vi "Save experiments in PGserver.vi"(6 "Param row name1":string="N", 7 "conninfo":T1={"host"="localhost", "port"="5432", "client_encoding"="WIN1251", "dbname"="system", "user"="postgres", "password"=""}, 8 "error in (no error)":errorcluster, 9 "Param column Name":string="value", 10 "Param Table":string="experiments", 11 "Parameter":string) -> (0 "error out":errorcluster)   [LabVIEW 2019]
uses:
  ctl/Coninfo.ctl
  PostgreSQL2LabVIEW/libpqlv/src/PQresultErrorMessage.vi
  PostgreSQL2LabVIEW/libpqUtility/src/PQclear.vi
  PostgreSQL2LabVIEW/libpqlv/src/PQsendQuery.vi
  PostgreSQL2LabVIEW/libpqlv/src/PQgetResult.vi
  PostgreSQL2LabVIEW/libpqlv/src/PQresultStatus.vi
  PostgreSQL2LabVIEW/libpqlv/src/PQfinish.vi
  PostgreSQL2LabVIEW/libpqlv/src/PQconnectdb.vi
  PostgreSQL2LabVIEW/libpqlv/src/PQerrorMessage.vi
  PostgreSQL2LabVIEW/libpqlv/src/PQstatus.vi
  <vilib>/dlg_ctls.llb/Space Constant.vi
  PostgreSQL2LabVIEW/libpqlv/src/PQclear.vi
  PostgreSQL2LabVIEW/libpqUtility/libpqutility.lvlib
  PostgreSQL2LabVIEW/libpqUtility64/libpqutility64.lvlib
  PostgreSQL.lvlib
panel:
  out "PQStatus":T2(ring)
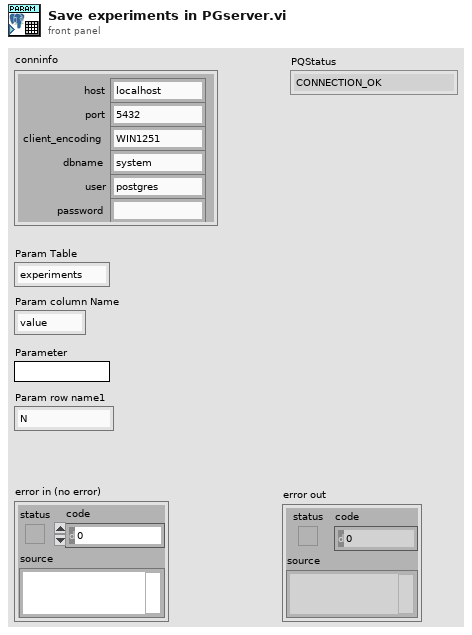
[diagram p1: front panel]
types:
  T1 = typedef "PostgreSQL.lvlib/Coninfo.ctl" = cluster{"host":string, "port":string, "client_encoding":string, "dbname":string, "user":string, "password":string}
  T2 = enum32{"CONNECTION_OK", "CONNECTION_BAD", "CONNECTION_STARTED", "CONNECTION_MADE", "CONNECTION_AWAITING_RESPONSE", "CONNECTION_AUTH_OK", "CONNECTION_SETENV", "CONNECTION_SSL_STARTUP", "CONNECTION_NEEDED"}
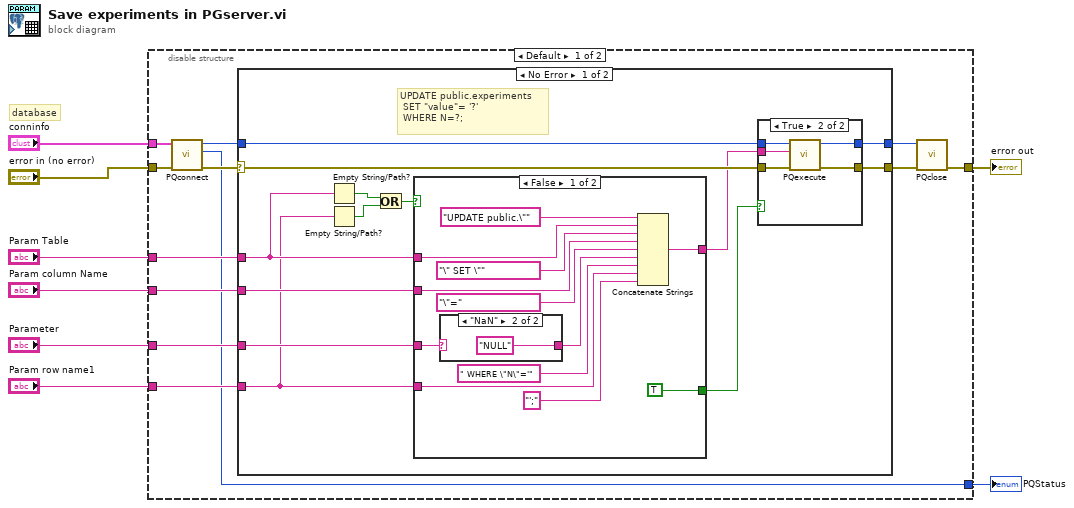
[diagram p0: block diagram]
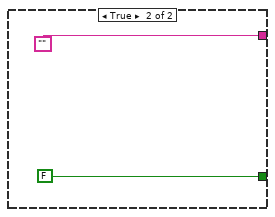
[diagram p3: hidden frame]
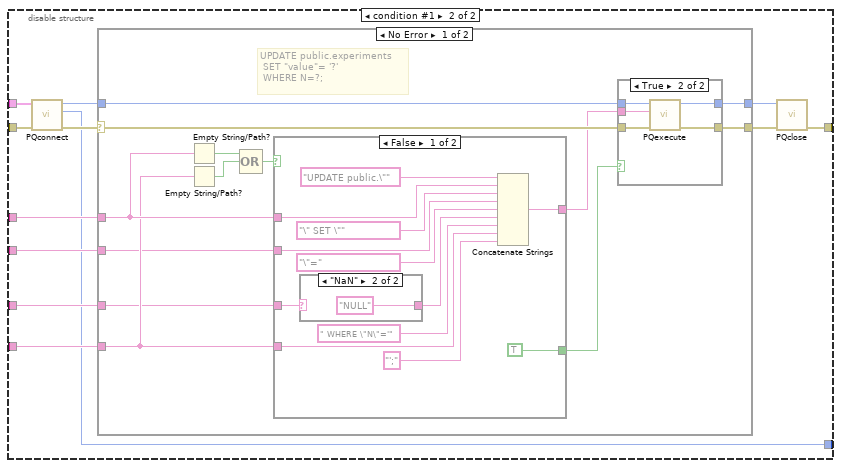
[diagram p6: hidden frame]
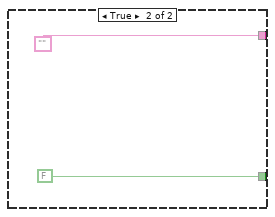
[diagram p8: hidden frame]
diagram:
  # "database"
  n1 = disable-structure shown="Default" {
    disable-tunnel: "Parameter" -> [w18 w62]
    disable-tunnel: [w16 w59] -> w7
    disable-tunnel: "conninfo" -> [w15 w66]
    disable-tunnel: "Param row name1" -> [w13 w61]
    disable-tunnel: "Param Table" -> [w12 w64]
    disable-tunnel: "Param column Name" -> [w11 w63]
    disable-tunnel: "error in (no error)" -> [w10 w65]
    disable-tunnel: [w9 w60] -> w1
    frame condition #0 (active) {
      n2 = call "PQconnect.vi"("error in (no error)"=w10, "conninfo"=w15) -> ("error out"=w20:errorcluster, "PQStatus"=w9:T2, "conn"=w19:u32)  [unwired: 7 in]
      n3 = case shown="No Error" w20 {
        selector: w20 -> [w33 w58]
        tunnel: w18 -> [w27 _]
        tunnel: w19 -> [w32 w57]
        tunnel: w12 -> [w25 _]
        tunnel: [w31 w58] -> w14
        tunnel: w13 -> [w23 _]
        tunnel: w11 -> [w26 _]
        tunnel: [w28 w57] -> w17
        frame No Error {
          # "UPDATE public.experiments\n\tSET \"value\"= '?'\n\tWHERE N=?;"
          n4 = Empty String/Path?(string/path=w25) -> (empty?=w30:bool)
          n5 = Empty String/Path?(string/path=w23) -> (empty?=w29:bool)
          n6 = Or(x=w30, y=w29) -> (x .or. y?=w24:bool)
          n7 = case shown="False" w24 {
            tunnel: [w44 ""] -> w21
            tunnel: w25 -> [w42 _]
            tunnel: [TRUE FALSE] -> w22
            tunnel: w23 -> [w37 _]
            tunnel: w27 -> [w36 _]
            tunnel: w26 -> [w39 _]
            frame False {
              n8 = case shown="\"NaN\"" w36 {
                selector: w36 -> [w46 _]
                tunnel: [w46 "NULL"] -> w35
                frame "", Default {
                }
                frame "NaN" {
                }
              }
              n9 = Concatenate Strings("UPDATE public.\"" ("table"), w42, "\" SET \"" ("table"), w39, "\"=" ("table"), w35, " WHERE \"N\"='" ("string"), w37, "';" ("string")) -> (w44:string)
            }
            frame True {
            }
          }
          n10 = case shown="True" w22 {
            tunnel: w33 -> [w51 w56]
            tunnel: w32 -> [w50 w54]
            tunnel: w21 -> [_ w55]
            tunnel: [w51 w53] -> w31
            tunnel: [w50 w52] -> w28
            frame False {
            }
            frame True {
              n11 = call "PQexecute.vi"("error in"=w56, "SQL querry"=w55, "conn"=w54) -> ("error out"=w53:errorcluster, "conn_out"=w52:u32)  [unwired: 7 in]
            }
          }
        }
        frame Error {
        }
      }
      n12 = call "PQclose.vi"("error in (no error)"=w14, "conn"=w17) -> ("error out"=w16:errorcluster)  [unwired: 9 in]
    }
    frame condition #1 {
      n13 = call "PQconnect.vi"("error in (no error)"=w65, "conninfo"=w66) -> ("error out"=w70:errorcluster, "PQStatus"=w60:T2, "conn"=w69:u64)  [unwired: 7 in]
      n14 = case shown="No Error" w70 {
        selector: w70 -> [w83 w108]
        tunnel: w62 -> [w74 _]
        tunnel: w69 -> [w82 w107]
        tunnel: w64 -> [w77 _]
        tunnel: [w81 w108] -> w67
        tunnel: w61 -> [w75 _]
        tunnel: w63 -> [w73 _]
        tunnel: [w78 w107] -> w68
        frame No Error {
          # "UPDATE public.experiments\n\tSET \"value\"= '?'\n\tWHERE N=?;"
          n15 = Empty String/Path?(string/path=w77) -> (empty?=w80:bool)
          n16 = Empty String/Path?(string/path=w75) -> (empty?=w79:bool)
          n17 = Compound Arithmetic op=OR(w80, w79) -> (w76:bool)  [unwired: 1 in]
          n18 = case shown="False" w76 {
            tunnel: [w94 ""] -> w71
            tunnel: w77 -> [w92 _]
            tunnel: [TRUE FALSE] -> w72
            tunnel: w75 -> [w87 _]
            tunnel: w74 -> [w86 _]
            tunnel: w73 -> [w89 _]
            frame False {
              n19 = case shown="\"NaN\"" w86 {
                selector: w86 -> [w96 _]
                tunnel: [w96 "NULL"] -> w85
                frame "", Default {
                }
                frame "NaN" {
                }
              }
              n20 = Concatenate Strings("UPDATE public.\"" ("table"), w92, "\" SET \"" ("table"), w89, "\"=" ("table"), w85, " WHERE \"N\"='" ("string"), w87, "';" ("string")) -> (w94:string)
            }
            frame True {
            }
          }
          n21 = case shown="True" w72 {
            tunnel: w83 -> [w101 w106]
            tunnel: w82 -> [w100 w104]
            tunnel: w71 -> [_ w105]
            tunnel: [w101 w103] -> w81
            tunnel: [w100 w102] -> w78
            frame False {
            }
            frame True {
              n22 = call "PQexecute.vi"("error in"=w106, "SQL querry"=w105, "conn"=w104) -> ("error out"=w103:errorcluster, "conn_out"=w102:u64)  [unwired: 7 in]
            }
          }
        }
        frame Error {
        }
      }
      n23 = call "PQclose.vi"("error in (no error)"=w67, "conn"=w68) -> ("error out"=w59:errorcluster)  [unwired: 9 in]
    }
  }
  "error out" <- w7
  "PQStatus" <- w1
